vi "Setup Printing.vi"(11 "error in (no error)":errorcluster) -> (15 "error out":errorcluster)   [LabVIEW 2014, in "lvprj2html.lvlib"]
uses:
  lvprj2html.lvlib
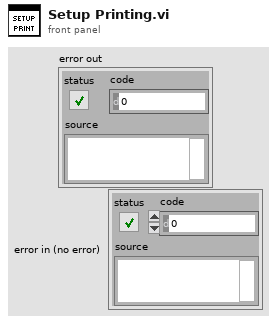
[diagram p1: front panel]
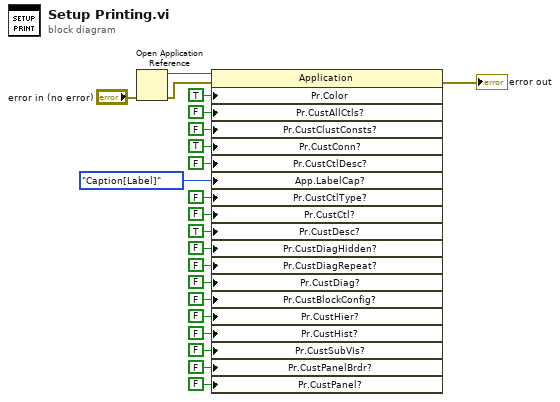
[diagram p0: block diagram]
diagram:
  n1 = Open Application Reference(8:"error in (no error)") -> (0:w2:errorcluster, 3:w3:refnum<vi>)  [unwired: 3 in]
  n2 = property class="Application"(reference=w3, error in=w2, "Pr.Color"=TRUE ("Printing:Color/Grayscale?"), "Pr.CustAllCtls?"=FALSE ("Printing:Custom All Controls?"), "Pr.CustClustConsts?"=FALSE ("Printing:Custom Cluster Constants?"), "Pr.CustConn?"=TRUE ("Printing:Custom Connector?"), "Pr.CustCtlDesc?"=FALSE ("Printing:Custom Control Descriptions?"), "App.LabelCap?"=enum16{"Label", "Caption", "Caption[Label]"}."Caption[Label]" ("Printing:Custom Control Label/Caption?"), "Pr.CustCtlType?"=FALSE ("Printing:Custom Control Types?"), "Pr.CustCtl?"=FALSE ("Printing:Custom Controls?"), "Pr.CustDesc?"=TRUE ("Printing:Custom Description?"), "Pr.CustDiagHidden?"=FALSE ("Printing:Custom Diagram Hidden?"), "Pr.CustDiagRepeat?"=FALSE ("Printing:Custom Diagram Repeat?"), "Pr.CustDiag?"=FALSE ("Printing:Custom Diagram?"), "Pr.CustBlockConfig?"=FALSE ("Printing:Custom Express VI Configuration?"), "Pr.CustHier?"=FALSE ("Printing:Custom Hierarchy?"), "Pr.CustHist?"=FALSE ("Printing:Custom History?"), "Pr.CustSubVIs?"=FALSE ("Printing:Custom List of SubVIs?"), "Pr.CustPanelBrdr?"=FALSE ("Printing:Custom Panel Border?"), "Pr.CustPanel?"=FALSE ("Printing:Custom Panel?")) -> (error out=→"error out":errorcluster)  [unwired: 1 out]
